vi "Static Read.vi"(8 "error in (no error)":errorcluster, 11 "Abs_Double Float in":refnum<class "Abs_Complex Single Float 1D.lvclass">) -> (0 "error out":errorcluster, 2 "Value":T1, 3 "Abs_Double Float out":refnum<class "Abs_Complex Single Float 1D.lvclass">)   [LabVIEW 2021, in "Abs_Complex Single Float 1D.lvclass"]
uses:
  Abs_Complex Single Float 1D.lvclass
  Support/Type.ctl
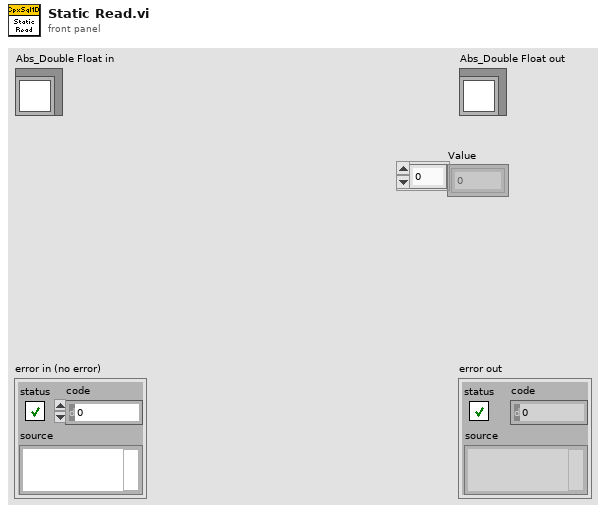
[diagram p1: front panel]
types:
  T1 = typedef "Abs_Complex Single Float 1D.lvclass/Type.ctl" = csg[]
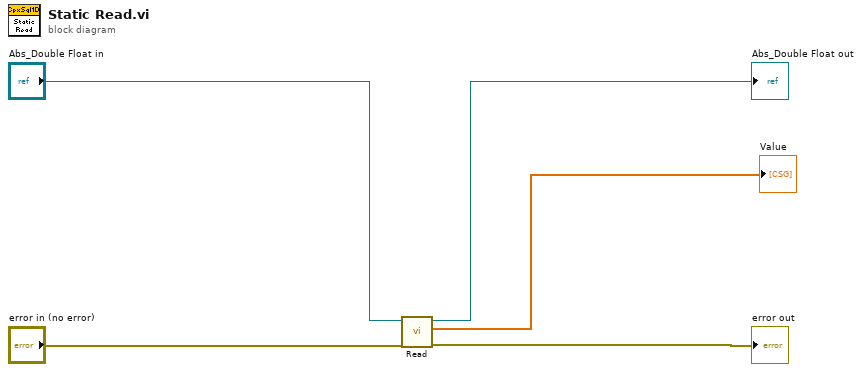
[diagram p0: block diagram]
diagram:
  n1 = call-dynamic "Read.vi"("error in (no error)"="error in (no error)", "Double Float.lvclass_340760 in"="Abs_Double Float in") -> ("error out"=→"error out":errorcluster, "Value"=→"Value":T1, "Double Float.lvclass_340760 out"=→"Abs_Double Float out":refnum<class "Abs_Complex Single Float 1D.lvclass">)  [unwired: 7 in]
